vi "Page_Destination_Initialize.vi"(8 "error in (no error)":errorcluster, 9 "ctlReferences":T1, 11 "Build in":refnum<class "AB_Build.lvclass">) -> (0 "error out":errorcluster, 3 "Build out":refnum<class "AB_Build.lvclass">)   [LabVIEW 2020, in "AB_Deployment.lvlib"]
uses:
  <vilib>/AppBuilder/AB_Classes/Deployment/AB_Deployment.lvlib
  <vilib>/AppBuilder/AB_Classes/Build/AB_Build.lvclass
  <resource>/Framework/Providers/Builds/AppBuilder/AB_UI_Page_Destination_References.ctl
  <resource>/Framework/Providers/Common/provcom_StringGlobals.vi
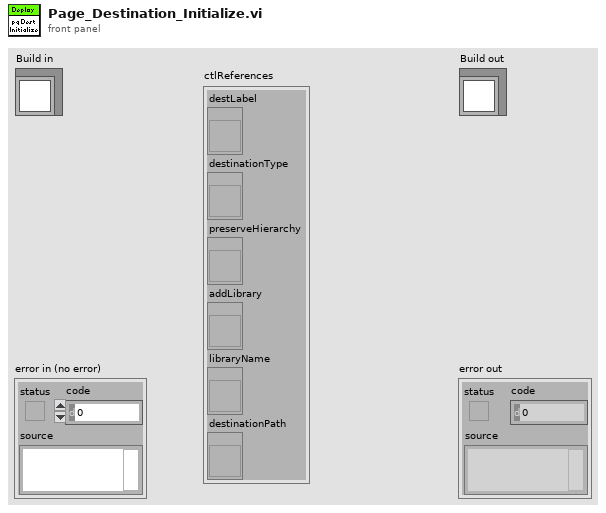
[diagram p1: front panel]
types:
  T1 = typedef "AB_UI_Page_Destination_References.ctl" = cluster{"destLabel":refnum<vi>, "destinationType":refnum<vi>, "preserveHierarchy":refnum<vi>, "addLibrary":refnum<vi>, "libraryName":refnum<vi>, "destinationPath":refnum<vi>}
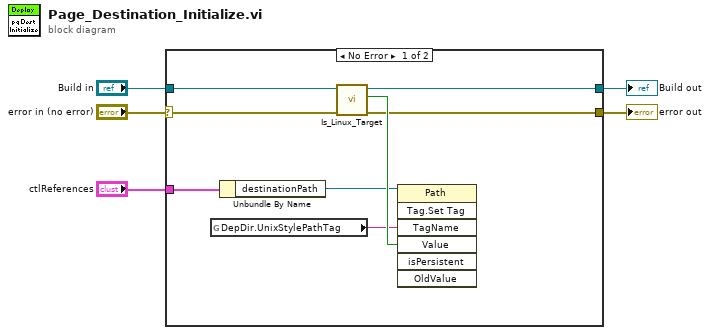
[diagram p0: block diagram]
diagram:
  n1 = case shown="No Error" "error in (no error)" {
    selector: "error in (no error)" -> [w13 w15]
    tunnel: [w10 w15] -> w4
    tunnel: [w11 w14] -> w3
    tunnel: "ctlReferences" -> [w9 _]
    tunnel: "Build in" -> [w6 w14]
    frame No Error {
      n2 = global read "provcom_StringGlobals.vi" "DepDir.UnixStylePathTag"() -> (w7:string)
      n3 = Unbundle By Name(w9) -> ("destinationPath"=w8:refnum<vi>)
      n4 = call <vilib>:"Is_Linux_Target.vi"("error in (no error)"=w13, "AB_Build in"=w6) -> ("error out"=w10:errorcluster, "Linux?"=w12:bool, "AB_Build out"=w11:refnum<class "AB_Build.lvclass">)  [unwired: 7 in]
      n5 = invoke class="Path" method="Tag.Set Tag"(reference=w8, "TagName"=w7, "Value"=w12) -> ()  [unwired: 4 in, 7 out]
    }
    frame Error {
    }
  }
  "error out" <- w4
  "Build out" <- w3
